vi "OPC Set Tag Name.vi"(7 "data type":T1=11 items=["Boolean"=1, "SByte"=2, "Byte"=3, "Int16"=4, "UInt16"=5, "Int32"=6, "UInt32"=7, "Int64"=8, "UInt64"=9, "Float"=10, "Double"=11, "String"=12, "DateTime"=13, "ByteString"=15, "Array of Boolean"=101, "Array of SByte"=102, "Array of Byte"=103, "Array of Int16"=104, "Array of UInt16"=105, "Array of Int32"=106, "Array of UInt32"=107, "Array of Int64"=108, "Array of UInt64"=109, "Array of Float"=110, "Array of Double"=111, "Array of String"=112, "Array of DateTime"=113, "Array of ByteString"=115, "Matrix of Boolean"=201, "Matrix of SByte"=202, "Matrix of Byte"=203, "Matrix of Int16"=204, "Matrix of UInt16"=205, "Matrix of Int32"=206, "Matrix of UInt32"=207, "Matrix of Int64"=208, "Matrix of UInt64"=209, "Matrix of Float"=210, "Matrix of Double"=211, "Matrix of String "=212, "Matrix of DateTime"=213, "Matrix of ByteString"=215], 8 "error in (no error)":errorcluster, 9 "name":string, 10 "item node ID":T2, 11 "Refnum in":T5) -> (0 "error out":errorcluster, 3 "OPC Property cluster":T4)   [LabVIEW 2018]
uses:
  <vilib>/OPCUA/controls/NodeId.ctl
  <vilib>/OPCUA/controls/OPC UA Server Refnum.ctl
  <vilib>/OPCUA/controls/OPC UA Variable Node Refnum.ctl
  <vilib>/OPCUA/controls/Data Type.ctl
  <vilib>/OPCUA/NI OPC UA Server.lvlib
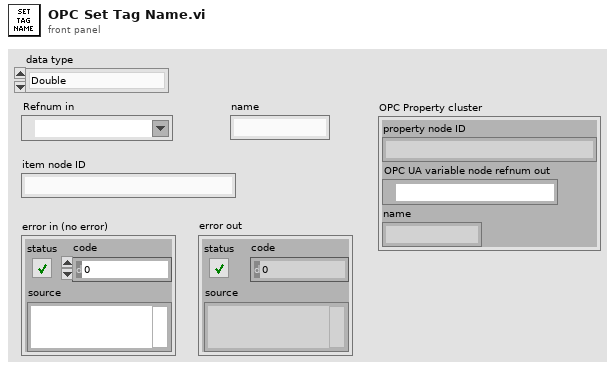
[diagram p1: front panel]
types:
  T1 = typedef "Data Type.ctl" = u16
  T2 = typedef "NodeId.ctl" = string
  T3 = typedef "OPC UA Variable Node Refnum.ctl" = refnum<k21>
  T4 = cluster{"property node ID":T2, "OPC UA variable node refnum out":T3, "name":string}
  T5 = typedef "OPC UA Server Refnum.ctl" = refnum<k21>
  T6 = cluster{"Tag ID":T2, "OPC UA variable node refnum out":T3, "name":string}
  T7 = cluster{"name":string, "data type":T1, "access level":u16, "description":string}
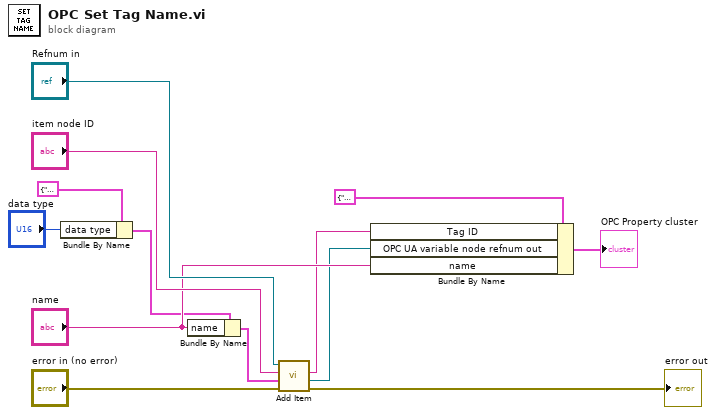
[diagram p0: block diagram]
diagram:
  n1 = Bundle By Name(cluster=T7 {"name"="", "data type"=11, "access level"=3, "description"=""} ("property"), "data type"="data type") -> (w2:T7)
  n2 = Bundle By Name(cluster=w2, "name"="name") -> (w7:T7)
  n3 = call <vilib>:"Add Item.vi"("error in (no error)"="error in (no error)", "item"=w7, "parent folder node ID"="item node ID", "OPC UA server refnum in"="Refnum in") -> ("error out"=→"error out":errorcluster, "OPC UA variable node refnum out"=w4:T3, "item node ID"=w5:T2)  [unwired: 3 in, 1 out]
  n4 = Bundle By Name(cluster=T6 {"Tag ID"="", "OPC UA variable node refnum out"="", "name"=""}, "Tag ID"=w5, "OPC UA variable node refnum out"=w4, "name"="name") -> (→"OPC Property cluster":T6)
